vi "Time Out.vi"(8 "error in (no error)":errorcluster={"status"=TRUE, "code"=5000, "source"="User hit cancel"}, 10 "?":string="Valves 1 and 2 venting to atmoshphere", 11 "Numeric":i32=40) -> (0 "error out":errorcluster={"status"=TRUE, "code"=5000, "source"="User hit cancel"})   [LabVIEW 2018]
panel:
  out "?":string="seconds remaining"
  out "?":i32=4
  in  "cancel":bool
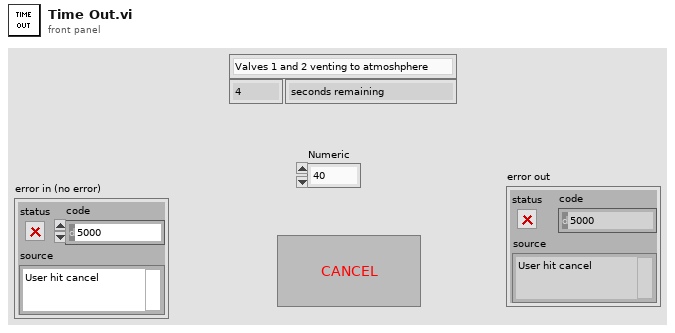
[diagram p1: front panel]
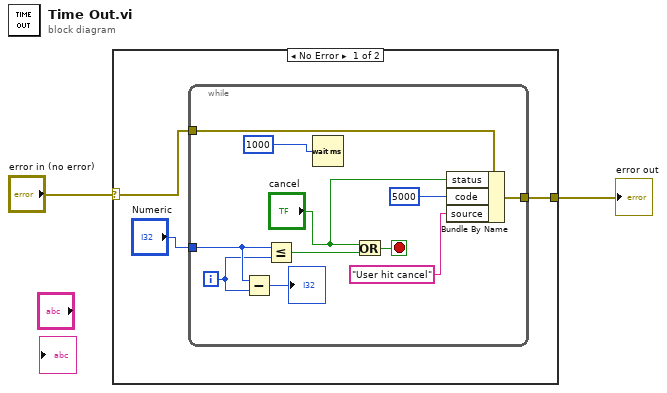
[diagram p0: block diagram]
diagram:
  n1 = case shown="No Error" "error in (no error)" {
    selector: "error in (no error)" -> [w4 w17]
    tunnel: [w3 w17] -> w1
    frame No Error {
      n2 = while {
        tunnel: "Numeric" -> [w12]
        tunnel: w4 -> [w9]
        tunnel: [w8] -> w3
        i -> [w11]
        stop <- w14 stop-if-true
        n3 = Subtract(x=w12, y=w11) -> (x-y=→"?":i32)
        n4 = Less Or Equal?(x=w12, y=w11) -> (x <= y?=w15:bool)
        n5 = Wait (ms)(milliseconds to wait=1000) -> ()  [unwired: 1 out]
        n6 = Or(x="cancel", y=w15) -> (x .or. y?=w14:bool)
        n7 = Bundle By Name(cluster=w9, "status"="cancel", "code"=5000, "source"="User hit cancel") -> (w8:errorcluster)
      }
    }
    frame Error {
    }
  }
  "error out" <- w1
